vi "dfd_Extension.vi"(8 "error in (no error)":errorcluster, 9 "extension length":i32, 10 "extension type":u16(ring) items=["zero padding", "symmetric", "periodic"], 11 "x[i]":dbl[](array[numeric]) format="%.2f") -> (0 "error out":errorcluster, 1 "final condition out":dbl[](array[numeric]) format="%.2f", 2 "x[i] dup.":dbl[](array[numeric]) format="%.2f", 3 "initial condition out":dbl[](array[numeric]) format="%.2f")   [LabVIEW 2017, in "NI_DigFilterLicensed.lvlib"]
uses:
  <vilib>/addons/Digital Filter Design/NI_DigFilterLicensed.lvlib
  <vilib>/addons/Digital Filter Design/_Misc.llb/dfd_Error Handlers (Single).vi
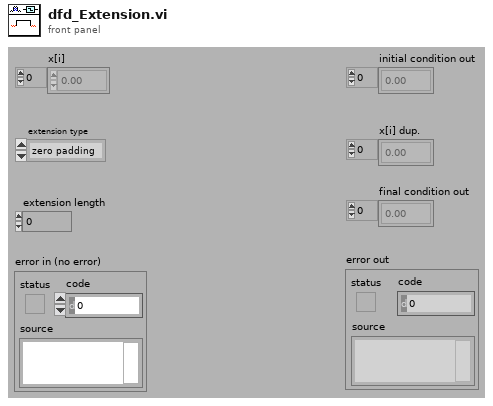
[diagram p1: front panel]
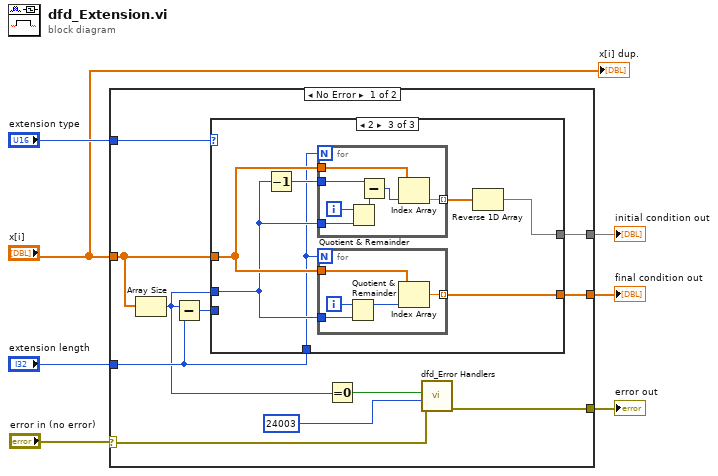
[diagram p0: block diagram]
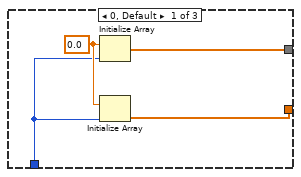
[diagram p2: hidden frame]
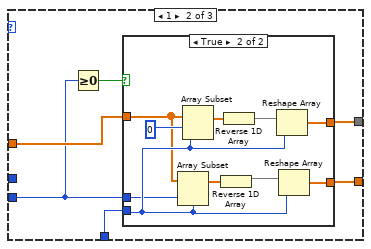
[diagram p3: hidden frame]
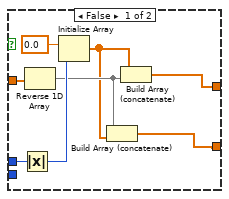
[diagram p4: hidden frame]
diagram:
  n1 = case shown="No Error" "error in (no error)" {
    selector: "error in (no error)" -> [w8 w66]
    tunnel: "extension type" -> [w18 _]
    tunnel: "extension length" -> [w17 _]
    tunnel: [w15 _] -> w5
    tunnel: [w14 _] -> w4
    tunnel: "x[i]" -> [w13 _]
    tunnel: [w9 w66] -> w2
    frame No Error {
      n2 = Array Size(array=w13) -> (size(s)=w12:i32)
      n3 = Subtract(x=w12, y=w17) -> (x-y=w16:i32)
      n4 = case shown="2" w18 {
        tunnel: w13 -> [_ w24 w52]
        tunnel: w17 -> [w21 w28 w49]
        tunnel: w16 -> [_ w23 _]
        tunnel: [w20 w25 w53] -> w14
        tunnel: [w19 w26 w47] -> w15
        tunnel: w12 -> [_ _ w51]
        frame 0, Default {
          w22 = 0.0
          n5 = Initialize Array(w22, w21) -> (w19:dbl[])
          n6 = Initialize Array(w22, w21) -> (w20:dbl[])
        }
        frame 1 {
          n7 = Greater Or Equal To 0?(x=w23) -> (x >= 0?=w27:bool)
          n8 = case shown="True" w27 {
            tunnel: [w32 w41] -> w26
            tunnel: [w29 w40] -> w25
            tunnel: w28 -> [_ w39]
            tunnel: w24 -> [w33 w38]
            tunnel: w23 -> [w36 w37]
            frame False {
              n9 = Absolute Value(x=w36) -> (abs(x)=w35:i32)
              n10 = Reverse 1D Array(array=w33) -> (reversed array=w31:dbl[])
              n11 = Initialize Array(0.0 ("element"), w35) -> (w30:dbl[])
              n12 = Build Array (concatenate)(w31, w30) -> (w29:dbl[])
              n13 = Build Array (concatenate)(w30, w31) -> (w32:dbl[])
            }
            frame True {
              n14 = Array Subset(array=w38, index=w37, length=w39) -> (w46:dbl[])
              n15 = Array Subset(array=w38, index=0, length=w39) -> (w45:dbl[])
              n16 = Reverse 1D Array(array=w46) -> (reversed array=w43:dbl[])
              n17 = Reverse 1D Array(array=w45) -> (reversed array=w42:dbl[])
              n18 = Reshape Array(w42, w39) -> (w41:dbl[])
              n19 = Reshape Array(w43, w39) -> (w40:dbl[])
            }
          }
        }
        frame 2 {
          n20 = Decrement(x=w51) -> (x-1=w50:i32)
          n21 = for {
            N: w49 -> [_]
            tunnel: w52 -> [w60]
            tunnel: [w59] -> w48 mode=indexing
            tunnel: w51 -> [w58]
            tunnel: w50 -> [w55]
            i -> [w57]
            n22 = Quotient & Remainder(x=w57, y=w58) -> (x-y*floor(x/y)=w56:i32)  [unwired: 1 out]
            n23 = Subtract(x=w55, y=w56) -> (x-y=w54:i32)
            n24 = Index Array(array=w60, index=w54) -> (element=w59:dbl)
          }
          n25 = for {
            N: w49 -> [_]
            tunnel: w52 -> [w65]
            tunnel: [w64] -> w53 mode=indexing
            tunnel: w51 -> [w62]
            i -> [w63]
            n26 = Quotient & Remainder(x=w63, y=w62) -> (x-y*floor(x/y)=w61:i32)  [unwired: 1 out]
            n27 = Index Array(array=w65, index=w61) -> (element=w64:dbl)
          }
          n28 = Reverse 1D Array(array=w48) -> (reversed array=w47:dbl[])
        }
      }
      n29 = Equal To 0?(x=w12) -> (x = 0?=w11:bool)
      n30 = call-poly <vilib>:"dfd_Error Handlers.vi"("error in (no error)"=w8, "error code"=24003 ("WRN_#INPUT_ZERO"), "condition failed?"=w11) -> ("error out"=w9:errorcluster)  [unwired: 8 out]
    }
    frame Error {
    }
  }
  "initial condition out" <- w5
  "final condition out" <- w4
  "error out" <- w2
  "x[i] dup." <- "x[i]"
